vi "USB4704 #2 Buffered AI V10.1vi.vi"() -> ()   [LabVIEW 2013]
uses:
  <vilib>/Platform/TimedLoop/XDataNode/timing_clust.ctl
  <vilib>/Platform/TimedLoop/XDataNode/nitl_modes.ctl
  <vilib>/Platform/TimedLoop/XDataNode/wakeup.ctl
  <userlib>/DAQNavi Polymorphic VI/create/DAQNavi Create Channel(AI-Voltage).vi
  <userlib>/DAQNavi Polymorphic VI/configure/timing/DAQNavi Timing(Convert Clock).vi
  <userlib>/DAQNavi Polymorphic VI/read/DAQNavi Read (Analog 1D Wfm NChan NSamp).vi
  <vilib>/platform/TimedLoop/XDataNode/XDataNode.xnode
  <vilib>/Platform/TimedLoop/XDataNode/XDNodeRunTimeDep.lvlib
panel:
  out "loop time":dbl
  out "error out":errorcluster
  out "Waveform Graph 2":waveform(dbl)[](graph)
  out "value range":string="+/- 5 V" caption="property value"
  in  "number of samples per channel to read":u32=1000
  in  "samples per channel":i32=1000
  in  "convert clock rate":dbl=1000.0
  out "physical channels":string="DemoDevice,BID#0/ai0:1" caption="property value"
  # "Please modify physical channels and value range in Channel Parameters\nthrough DAQNavi Property Assistant VI  in block diagram."
  # "Channel Parameters"
  # "Timing Parameters"
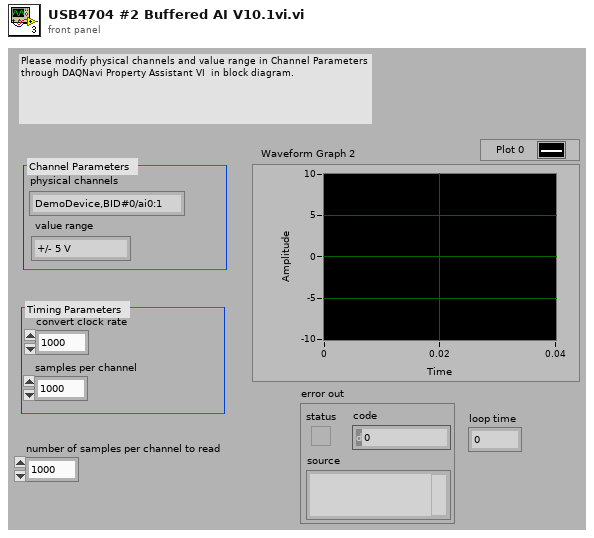
[diagram p1: front panel]
types:
  T1 = typedef "XDNodeRunTimeDep.lvlib/timing_clust.ctl" = cluster{"Expected End [f-1]":u64, "Actual End [f-1]":u64, "Finished Late? [f-1]":bool, "Expected End [i-1]":u64, "Actual End [i-1]":u64, "Finished Late? [i-1]":bool, "Expected Start [i]":u64, "Actual Start [i]":u64, "Expected Start [f]":u64, "Actual Start [f]":u64, "Source Name":string, "Structure Name":string, "Period":i64, "Deadline":i64, "Offset":i64, "Start":i64, "Priority":i32, "Timeout":i32, "Mode":T2, "Wakeup Reason":T3, "Error":errorcluster, "Source Type":string, "Secondary Source Type":string, "Global End Time":u64, "Global Start Time":u64, "Frame Duration":u64, "Iteration Duration":u64, "Assigned CPU":i32, "I/O Scan Engine Mode":u32}
  T2 = typedef "XDNodeRunTimeDep.lvlib/nitl_modes.ctl" = enum32{"No Change", "Process missed periods, maintain original phase", "Discard missed periods, maintain original phase", "Process missed periods, ignore original phase", "Discard missed periods, ignore original phase"}
  T3 = typedef "XDNodeRunTimeDep.lvlib/wakeup.ctl" = enum32{"Normal", "Aborted", "Asynchronous wakeup", "Timing source error", "Timed loop error", "Timeout"}
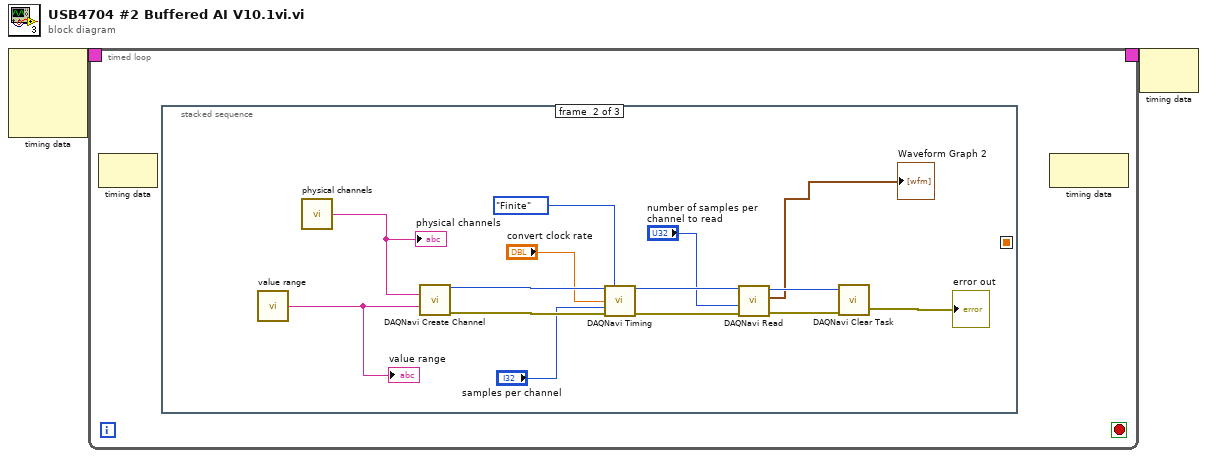
[diagram p0: block diagram]
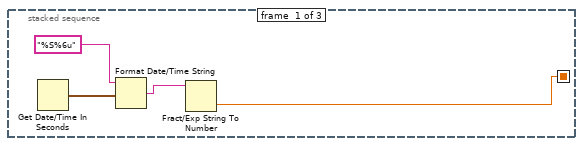
[diagram p2: hidden frame]
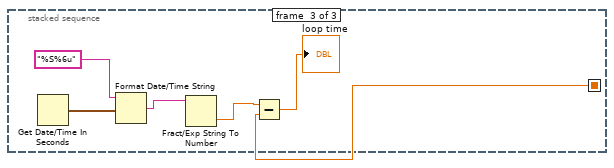
[diagram p3: hidden frame]
diagram:
  n1 = node-c288() -> (w2:T1)  [unwired: 4 in]
  n2 = timed-loop {
    timing: w2 -> [_]
    timing-out: [_] -> w1
    stop <- _ stop-if-true
    n3 = node-c288() -> ()  [unwired: 1 in, 1 out]
    n4 = stacked-sequence {
      seq-local: [w3 _ _] -> [_ _ w21]
      frame #0 {
        n5 = Get Date/Time In Seconds() -> (seconds since 1Jan1904=w5:timestamp)
        n6 = Format Date/Time String(time format string (%c)="%S%6u", seconds (now)=w5) -> (date/time string=w4:string)  [unwired: 1 in]
        n7 = Fract/Exp String To Number(string=w4) -> (number=w3:dbl)  [unwired: 3 in, 1 out]
      }
      frame #1 {
        n8 = call "value range"() -> ("property value"=w9:string)  [unwired: 1 out]
        "value range" <- w9
        n9 = call "physical channels"() -> ("property value"=w10:string)  [unwired: 1 out]
        "physical channels" <- w10
        n10 = call-poly <userlib>:"DAQNavi Create Channel.vi"("physical channels"=w10, "value range"=w9) -> ("task out"=w18:i32, "error out"=w17:errorcluster)  [unwired: 3 in, 9 out]
        n11 = call-poly <userlib>:"DAQNavi Timing.vi"("task in"=w18, "sample mode"=enum16{"Finite", "Continuous"}."Finite", "rate"="convert clock rate", "samples per channel"="samples per channel", "error in (no error)"=w17) -> ("task out"=w16:i32, "error out"=w15:errorcluster)  [unwired: 1 in, 8 out]
        n12 = call-poly <userlib>:"DAQNavi Read.vi"("error in (no error)"=w15, "number of samples per channel to read"="number of samples per channel to read", "task in"=w16) -> ("error out"=w19:errorcluster, "data"=→"Waveform Graph 2":waveform(dbl)[], "task out"=w20:i32)  [unwired: 1 in, 5 out]
        n13 = call <userlib>:"DAQNavi Clear Task.vi"("error in (no error)"=w19, "task in"=w20) -> ("error out"=→"error out":errorcluster)  [unwired: 1 out]
      }
      frame #2 {
        n14 = Get Date/Time In Seconds() -> (seconds since 1Jan1904=w25:timestamp)
        n15 = Format Date/Time String(time format string (%c)="%S%6u", seconds (now)=w25) -> (date/time string=w24:string)  [unwired: 1 in]
        n16 = Fract/Exp String To Number(string=w24) -> (number=w23:dbl)  [unwired: 3 in, 1 out]
        n17 = Subtract(x=w23, y=w21) -> (x-y=→"loop time":dbl)
      }
    }
    n18 = node-c288() -> ()  [unwired: 1 in, 1 out]
  }
  n19 = node-c288(w1) -> ()  [unwired: 1 out]
